vi "NewChannelsName.vi"(8 "error in (no error)":errorcluster) -> (0 "error out":errorcluster, 1 "通道数：":i32, 2 "Confirm":bool, 3 "AutoChls":T1(array[cluster]))   [LabVIEW 2015, in "Batch-Import-User-Channels Custom Device.lvlib"]
doc: "Displays a standard dialog box that prompts users to enter information, such as a user name and password.\n--------------------\n\nThis Express VI is configured as follows:\n\nMessage to Display to the User:\nThe inputs are: \nText Entry Box: Auto Channels"
uses:
  Batch-Import-User-Channels Custom Device.lvlib
  <vilib>/Utility/config.llb/Read Key (String).vi
  <vilib>/Utility/config.llb/NI_LVConfig.lvlib
panel:
  in  "Path":path
  in  "Cancel":bool
  in  "OK":bool
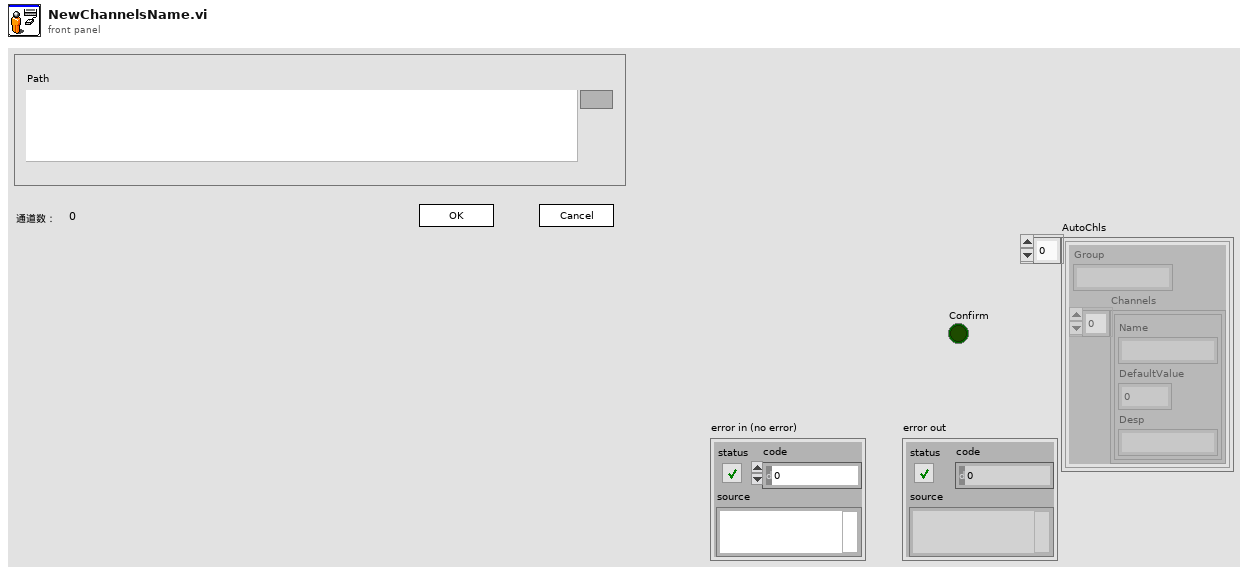
[diagram p1: front panel]
types:
  T1 = cluster{"Group":string, "Channels":cluster{"Name":string, "DefaultValue":dbl, "Desp":string}[]}[]
  T2 = enum32{"Invalid", "Standard", "Closed", "Hidden", "Minimized", "Maximized"}
  T3 = cluster{"Group":string, "Channels":cluster{"Name":string, "DefaultValue":dbl, "Desp":string}[]}
  T4 = cluster{"Name":string, "DefaultValue":dbl, "Desp":string}
  T5 = typedef "NI_LVConfig.lvlib/Config Data RefNum.ctl" = refnum<k1>
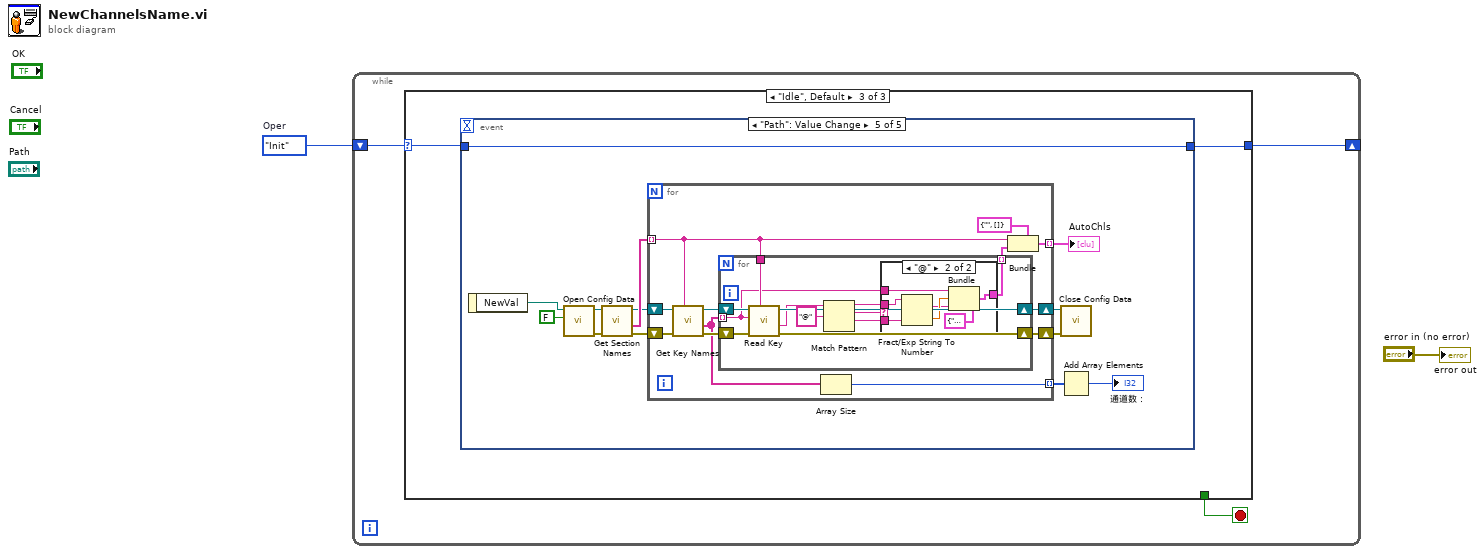
[diagram p0: block diagram]
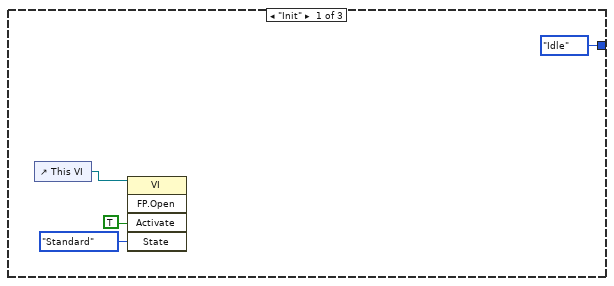
[diagram p2: hidden frame]
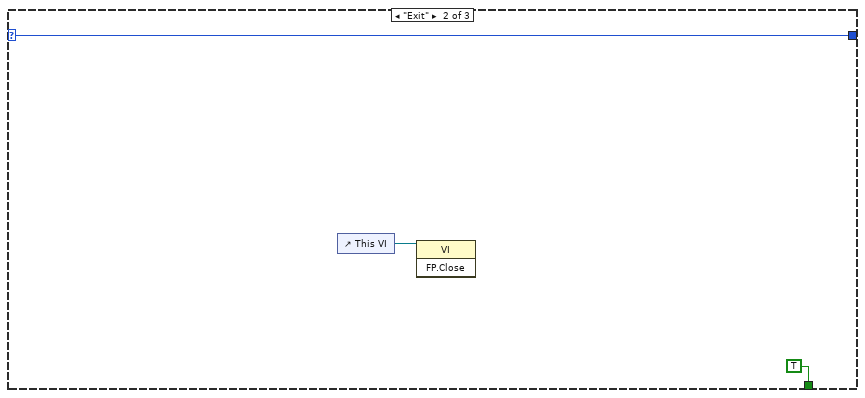
[diagram p3: hidden frame]
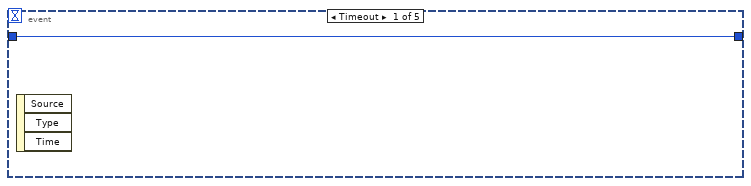
[diagram p4: hidden frame]
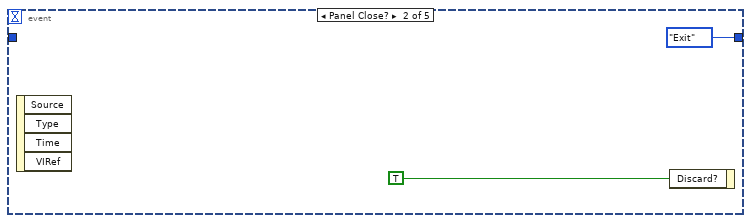
[diagram p5: hidden frame]
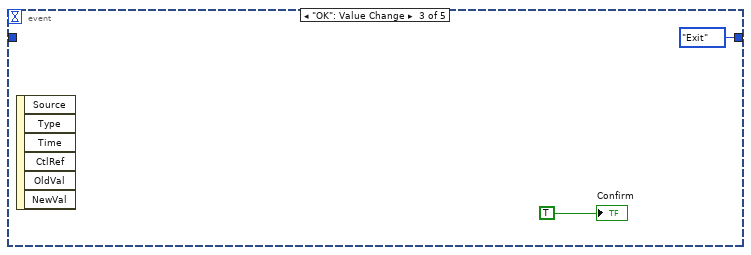
[diagram p6: hidden frame]
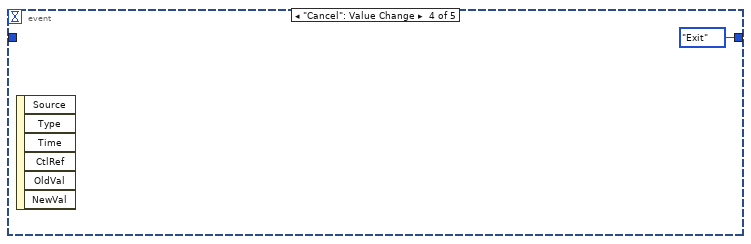
[diagram p7: hidden frame]
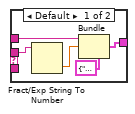
[diagram p8: hidden frame]
diagram:
  w2 = enum16{"Idle", "Init", "Exit"}."Init"  # Oper
  n1 = while {
    shift-right: [w5] -> _
    shift-left: w2 -> [w4]
    stop <- w3 stop-if-true
    n2 = case shown="\"Idle\", Default" w4 {
      selector: w4 -> [_ w12 w14]
      tunnel: [enum16{"Idle", "Init", "Exit"}."Idle" ("Oper") w12 w13] -> w5
      tunnel: [_ TRUE _] -> w3
      frame "Init" {
        n3 = control-ref of="This VI"() -> (w7:refnum<vi>)
        n4 = invoke class="VI" method="FP.Open"(reference=w7, "Activate"=TRUE ("Activate?"), "State"=T2."Standard") -> ()  [unwired: 2 in, 5 out]
      }
      frame "Exit" {
        n5 = control-ref of="This VI"() -> (w10:refnum<vi>)
        n6 = invoke class="VI" method="FP.Close"(reference=w10) -> ()  [unwired: 2 in, 3 out]
      }
      frame "Idle", Default {
        n7 = event shown="[4] \"Path\": Value Change" {
          selector: _ -> [_ _ _ _ _]
          dyn-events: _ -> [_ _ _ _ _]
          timeout: _ -> [_ _ _ _ _]
          tunnel: w14 -> [w15 _ _ _ w33]
          tunnel: [w15 enum16{"Idle", "Init", "Exit"}."Exit" ("Oper") enum16{"Idle", "Init", "Exit"}."Exit" ("Oper") enum16{"Idle", "Init", "Exit"}."Exit" ("Oper") w33] -> w13
          event Timeout {
            n8 = event-data() -> ()  [unwired: 1 in, 3 out]
          }
          event Panel Close? {
            n9 = event-data() -> ()  [unwired: 1 in, 4 out]
            n10 = event-data("Discard?"=TRUE) -> ()  [unwired: 1 in, 1 out]
          }
          event "OK": Value Change {
            n11 = event-data() -> ()  [unwired: 1 in, 6 out]
            "Confirm" <- TRUE ("Confirm")
          }
          event "Cancel": Value Change {
            n12 = event-data() -> ()  [unwired: 1 in, 6 out]
          }
          event "Path": Value Change {
            n13 = event-data() -> ("NewVal"=w31:path)  [unwired: 1 in]
            n14 = call <vilib>:"Open Config Data.vi"("create file if necessary (T)"=FALSE, "configuration file path"=w31) -> ("error out"=w30:errorcluster, "refnum"=w29:T5)  [unwired: 7 in, 1 out]
            n15 = call <vilib>:"Get Section Names.vi"("error in (no error)"=w30, "refnum"=w29) -> ("error out"=w25:errorcluster, "section names"=w28:string[], "refnum out"=w27:T5)  [unwired: 7 in]
            n16 = for {
              tunnel: w28 -> [w39] mode=indexing
              shift-right: [w37] -> w26
              shift-left: w27 -> [w45]
              shift-right: [w38] -> w24
              shift-left: w25 -> [w44]
              tunnel: [w43] -> w23 mode=indexing
              tunnel: [w42] -> w21 mode=indexing
              n17 = call <vilib>:"Get Key Names.vi"("section"=w39, "error in (no error)"=w44, "refnum"=w45) -> ("error out"=w41:errorcluster, "key names"=w36:string[], "refnum out"=w40:T5)  [unwired: 5 in, 1 out]
              n18 = for {
                tunnel: w39 -> [w56]
                shift-right: [w55] -> w38
                shift-left: w41 -> [w57]
                shift-right: [w54] -> w37
                shift-left: w40 -> [w53]
                tunnel: w36 -> [w52] mode=indexing
                tunnel: [w51] -> w35 mode=indexing
                n19 = call-poly <vilib>:"Read Key.vi"("section"=w56, "error in (no error)"=w57, "key"=w52, "refnum"=w53) -> ("error out"=w55:errorcluster, "value"=w50:string, "refnum out"=w54:T5)  [unwired: 4 in, 1 out]
                n20 = Match Pattern(string=w50, regular expression="@") -> (before substring=w47:string, match substring=w48:string, after substring=w46:string)  [unwired: 1 in, 1 out]
                n21 = case shown="\"@\"" w48 {
                  tunnel: w52 -> [w61 w67]
                  tunnel: [w62 w68] -> w51
                  tunnel: w47 -> [w60 w66]
                  tunnel: w46 -> [_ w63]
                  frame Default {
                    n22 = Fract/Exp String To Number(string=w60) -> (number=w59:dbl)  [unwired: 3 in, 1 out]
                    n23 = Bundle(cluster=T4 {"Name"="", "DefaultValue"=0.0, "Desp"=""} ("Channel"), "Name"=w61, "DefaultValue"=w59) -> (w62:T4)  [unwired: 1 in]
                  }
                  frame "@" {
                    n24 = Fract/Exp String To Number(string=w66) -> (number=w65:dbl)  [unwired: 3 in, 1 out]
                    n25 = Bundle(cluster=T4 {"Name"="", "DefaultValue"=0.0, "Desp"=""} ("Channel"), "Name"=w67, "DefaultValue"=w65, "Desp"=w63) -> (w68:T4)
                  }
                }
              }
              n26 = Array Size(array=w36) -> (size(s)=w43:i32)
              n27 = Bundle(cluster=T3 {"Group"="", "Channels"=[]} ("Chl"), "Group"=w39, "Channels"=w35) -> (w42:T3)
            }
            "AutoChls" <- w21
            n28 = call <vilib>:"Close Config Data.vi"("error in (no error)"=w24, "refnum"=w26) -> ()  [unwired: 8 in, 2 out]
            n29 = Add Array Elements(numeric array=w23) -> (sum=→"通道数：":i32)
          }
        }
      }
    }
  }
  "error out" <- "error in (no error)"
